vi "Write Head Impulse Sheet.vi"(8 "error in (no error)":errorcluster, 10 "Head Impulse":refnum<class "Data Analyser Report.lvclass">, 11 "Excel Logger in":refnum<class "Excel Logger.lvclass">) -> (0 "error out":errorcluster, 3 "Excel Logger out":refnum<class "Excel Logger.lvclass">)   [LabVIEW 2014, in "Excel Logger.lvclass"]
uses:
  Excel Logger.lvclass
  Data Analyser Report/Data Analyser Report.lvclass
  Excel Logger.lvclass/Excel Logger.ctl
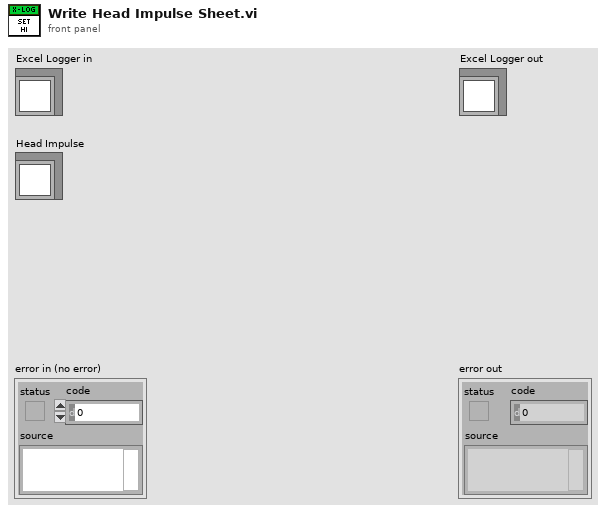
[diagram p1: front panel]
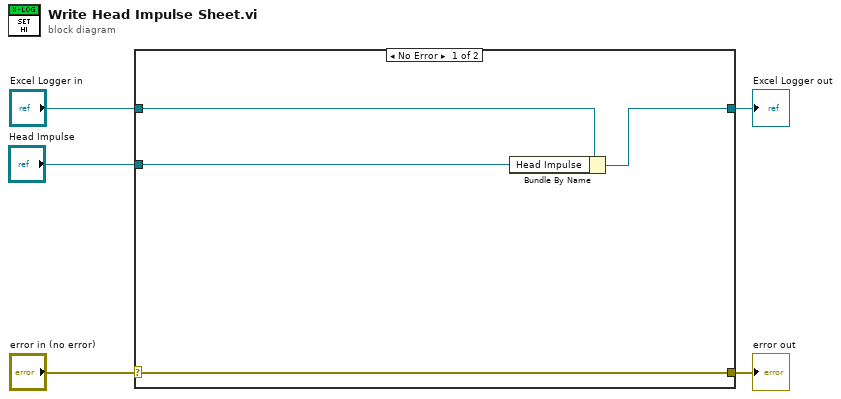
[diagram p0: block diagram]
diagram:
  n1 = case shown="No Error" "error in (no error)" {
    selector: "error in (no error)" -> [w9 w11]
    tunnel: [w9 w11] -> w4
    tunnel: [w8 w10] -> w2
    tunnel: "Excel Logger in" -> [w7 w10]
    tunnel: "Head Impulse" -> [w6 _]
    frame No Error {
      n2 = Bundle By Name(cluster=w7, "Head Impulse"=w6) -> (w8:refnum<class "Excel Logger.lvclass">)
    }
    frame Error {
    }
  }
  "error out" <- w4
  "Excel Logger out" <- w2
